vi "Read Holding Registers.vi"(7 "unit ID":u8, 8 "error in":errorcluster, 9 "number of inputs":u16, 10 "starting address":u16, 11 "Modbus slave in":refnum<class "Modbus Slave.lvclass">) -> (0 "error out":errorcluster, 2 "register values":u16[](array[numeric]), 3 "Modbus slave out":refnum<class "Modbus Slave.lvclass">)   [LabVIEW 2013, in "Modbus Library - Advance.lvlib" / "Modbus Slave.lvclass"]
doc: "Reads <B>number of inputs</B> holding registers starting at <B>starting address</B> from the device."
uses:
  Modbus Slave.lvclass
  Modbus Slave.lvclass/Modbus Slave.ctl
  Standard Data Model/Standard Data Model.lvclass
  Super Data Model/Super Data Model.lvclass
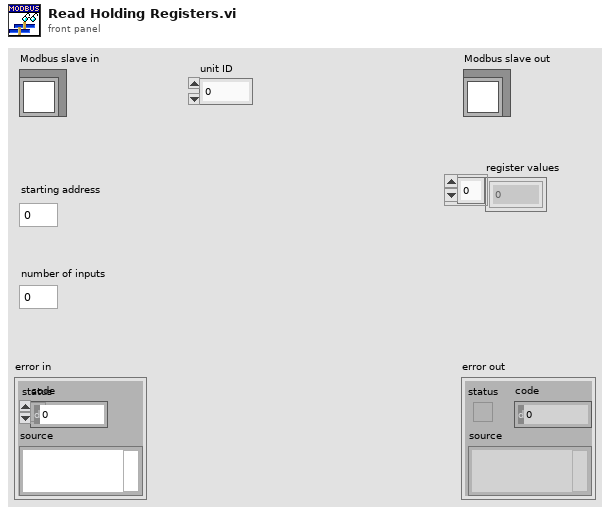
[diagram p1: front panel]
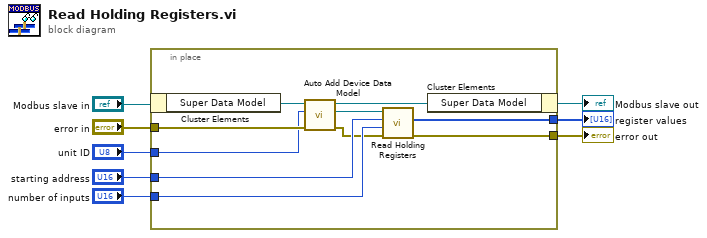
[diagram p0: block diagram]
diagram:
  n1 = in-place {
    in-place-border: [w10] -> w1
    in-place-border: "number of inputs" -> [w12]
    in-place-border: "starting address" -> [w13]
    in-place-border: [w11] -> w7
    in-place-border: "error in" -> [w17]
    in-place-border: "unit ID" -> [w15]
    n2 = in-place-cluster #1("Modbus slave in") -> ("Super Data Model"=w18:refnum<class "Super Data Model.lvclass">)
    n3 = call "Auto Add Device Data Model.vi"("error in"=w17, "unit ID"=w15, "Super Data Model in"=w18) -> ("error out"=w9:errorcluster, "device data model"=w14:refnum<class "Standard Data Model.lvclass">, "Super Data Model out"=w16:refnum<class "Super Data Model.lvclass">)  [unwired: 6 in]
    n4 = call-dynamic "Read Holding Registers.vi"("error in"=w9, "number of registers"=w12, "starting address"=w13, "Standard Data Model in"=w14) -> ("error out"=w11:errorcluster, "data"=w10:u16[])  [unwired: 5 in, 1 out]
    n5 = in-place-cluster #1("Super Data Model"=w16) -> (→"Modbus slave out":refnum<class "Modbus Slave.lvclass">)
  }
  "error out" <- w7
  "register values" <- w1
